vi "Detect Zero Crossing with Noise Threshold.vi"(7 "Noise Threshold":fxp<+/-,16,2>, 8 "Input Valid":bool=TRUE, 10 "x[n-1]":fxp<+/-,16,2>, 11 "x[n]":fxp<+/-,16,2>) -> (0 "Output Valid":bool=TRUE, 1 "zero crossing?":bool, 2 "x[n-1]":fxp<+/-,16,2> format="%.15g", 3 "x[n]":fxp<+/-,16,2> format="%.15g")   [LabVIEW 2011]
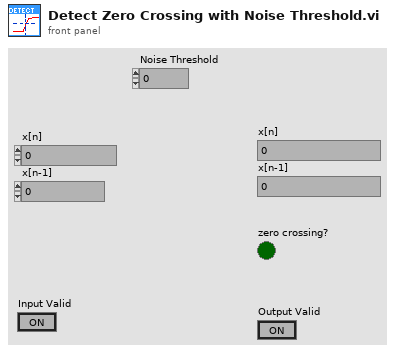
[diagram p1: front panel]
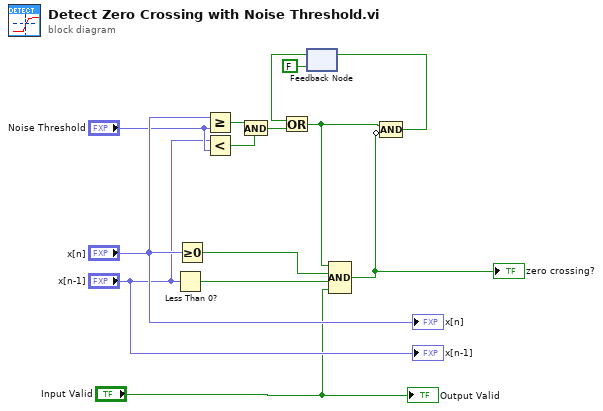
[diagram p0: block diagram]
diagram:
  n1 = Less Than 0?(x="x[n-1]") -> (x < 0?=w13:bool)
  n2 = Greater Or Equal To 0?(x="x[n]") -> (x >= 0?=w14:bool)
  n3 = Greater Or Equal?(x="x[n]", y="Noise Threshold") -> (x >= y?=w10:bool)
  n4 = Less?(x="x[n-1]", y="Noise Threshold") -> (x < y?=w9:bool)
  n5 = And(x=w10, y=w9) -> (x .and. y?=w8:bool)
  n6 = feedback #1(FALSE) -> (w4:bool)
  n7 = Or(x=w4, y=w8) -> (x .or. y?=w7:bool)
  n8 = Compound Arithmetic op=AND(w7, w14, w13, "Input Valid") -> (w6:bool)
  "zero crossing?" <- w6
  n9 = Compound Arithmetic op=AND(w7, invert w6) -> (w5:bool)
  n10 = feedback-in #1(w5) -> ()
  "x[n]" <- "x[n]"
  "x[n-1]" <- "x[n-1]"
  "Output Valid" <- "Input Valid"
